vi "Disconnect Channels (Multiple).vi"(8 "error in (no error)":errorcluster, 10 "disconnection list":string, 11 "SLSC Switch in":refnum<class "SLSC Switch.lvclass">) -> (0 "error out":errorcluster, 3 "SLSC Switch out":refnum<class "SLSC Switch.lvclass">)   [LabVIEW 2015, in "SLSC Switch.lvlib" / "SLSC Switch.lvclass"]
doc: "Breaks the connections between channels specified in disconnection list. If no connections exist between channels, SLSC-SWITCH returns an error. In the event of an error, the VI stops at the point in the list where the error occurred."
uses:
  SLSC Switch.lvclass
  slscsl/slscsl.lvclass
  <vilib>/SLSC/SLSC.lvlib
  <vilib>/SLSC/Unflatten Names (String).vi
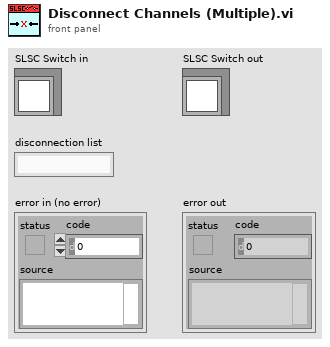
[diagram p1: front panel]
types:
  T1 = typedef "SLSC Switch.lvlib/slscsl.lvclass/SwitchActionsArray.ctl" = T2[]
  T2 = typedef "SLSC Switch.lvlib/slscsl.lvclass/SwitchAction.ctl" = cluster{"index":i32, "RelayAction":T3}
  T3 = typedef "SLSC Switch.lvlib/slscsl.lvclass/RelayAction.ctl" = u32
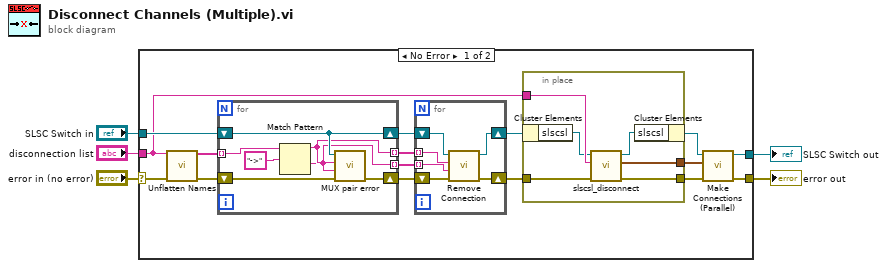
[diagram p0: block diagram]
diagram:
  n1 = case shown="No Error" "error in (no error)" {
    selector: "error in (no error)" -> [w7 w42]
    tunnel: [w11 w42] -> w4
    tunnel: "disconnection list" -> [w9 _]
    tunnel: "SLSC Switch in" -> [w18 w41]
    tunnel: [w12 w41] -> w2
    frame No Error {
      n2 = call-poly <vilib>:"Unflatten Names.vi"("names in"=w9, "error in (no error)"=w7) -> ("names out"=w8:string[], "error out"=w6:errorcluster)  [unwired: 12 in]
      n3 = for {
        tunnel: w8 -> [w27] mode=indexing
        shift-right: [w25] -> w17
        shift-left: w18 -> [w25]
        shift-right: [w22] -> w16
        shift-left: w6 -> [w26]
        tunnel: [w24] -> w15 mode=indexing
        tunnel: [w23] -> w14 mode=indexing
        n4 = Match Pattern(string=w27, regular expression="->") -> (before substring=w24:string, after substring=w23:string)  [unwired: 1 in, 2 out]
        n5 = call "MUX pair error.vi"("error in (no error)"=w26, "channel 2"=w23, "channel 1"=w24, "SLSC Switch in"=w25) -> ("error out"=w22:errorcluster)  [unwired: 7 in]
      }
      n6 = for {
        shift-right: [w33] -> w13
        shift-left: w17 -> [w34]
        shift-right: [w29] -> w10
        shift-left: w16 -> [w32]
        tunnel: w15 -> [w31] mode=indexing
        tunnel: w14 -> [w30] mode=indexing
        n7 = call "Remove Connection.vi"("error in (no error)"=w32, "channel 2"=w30, "channel 1"=w31, "SLSC Switch in"=w34) -> ("error out"=w29:errorcluster, "SLSC Switch out"=w33:refnum<class "SLSC Switch.lvclass">)  [unwired: 6 in]
      }
      n8 = in-place {
        in-place-border: w9 -> [w40]
        in-place-border: w10 -> [w39]
        in-place-border: [w38] -> w19
        in-place-border: [w35] -> w20
        n9 = in-place-cluster #1(w13) -> ("slscsl"=w37:refnum<class "slscsl.lvclass">)
        n10 = call "slscsl_disconnect.vi"("error in (no error)"=w39, "connectionList"=w40, "slscsl in"=w37) -> ("error out"=w38:errorcluster, "SwitchActionsArray"=w35:T1, "slscsl out"=w36:refnum<class "slscsl.lvclass">)  [unwired: 6 in]
        n11 = in-place-cluster #1("slscsl"=w36) -> (w21:refnum<class "SLSC Switch.lvclass">)
      }
      n12 = call "Make Connections (Parallel).vi"("error in (no error)"=w19, "switchActionsArray"=w20, "SLSC Switch in"=w21) -> ("error out"=w11:errorcluster, "SLSC Switch out"=w12:refnum<class "SLSC Switch.lvclass">)  [unwired: 7 in]
    }
    frame Error {
    }
  }
  "error out" <- w4
  "SLSC Switch out" <- w2
